vi "Byte Array to Supported Schemes.vi"(1 "Buffer":u8[](array[numeric])) -> (0 "Supported Schemes":T1[](array[typedef]))   [LabVIEW 2021, in "Field_RnD_Services_LIBSSH2_Toolkit.lvlib" / "Session.lvclass"]
doc: "Converts a byte array of comma-delimited string values into a list of supported authentication schemes by the remote SSH/SFTP server."
uses:
  Session.lvclass
  Session.lvclass/Session.ctl
  Type Definitions/User Authentication Schemes.ctl
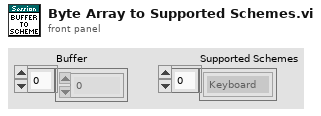
[diagram p1: front panel]
types:
  T1 = typedef "Field_RnD_Services_LIBSSH2_Toolkit.lvlib/Session.lvclass/User Authentication Schemes.ctl" = enum16{"Keyboard", "Password", "Public Key"}
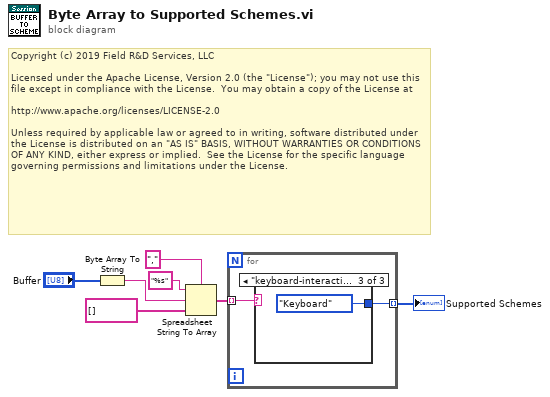
[diagram p0: block diagram]
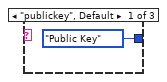
[diagram p2: hidden frame]
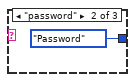
[diagram p3: hidden frame]
diagram:
  # "Copyright (c) 2019 Field R&D Services, LLC\n\nLicensed under the Apache License, Version 2.0 (the \"License\"); you may not use this file except in compliance with the License.  You may obtain a copy of the License at\n\nhttp://www.apache.org/licenses/LICENSE-2.0\n\nUnless required by applicable law or agreed to in writing, software distributed under the License is distributed on an \"AS IS\" BASIS, WITHOUT WARRANTIES OR CONDITIONS OF ANY KIND, either express or implied.  See the License for the specific language governing permissions and limitations under the License."
  n1 = Byte Array To String(unsigned byte array="Buffer") -> (string=w1:string)
  n2 = Spreadsheet String To Array(delimiter (Tab)=",", format string="%s", spreadsheet string=w1, array type (2D Dbl)=string[] []) -> (array=w5:string[])
  n3 = for {
    tunnel: w5 -> [w9] mode=indexing
    tunnel: [w8] -> w7 mode=indexing
    n4 = case shown="\"keyboard-interactive\"" w9 {
      tunnel: [User_Authentication_Schemes."Public Key" ("Scheme") User_Authentication_Schemes."Password" ("Scheme") User_Authentication_Schemes."Keyboard" ("Scheme")] -> w8
      frame "publickey", Default {
      }
      frame "password" {
      }
      frame "keyboard-interactive" {
      }
    }
  }
  "Supported Schemes" <- w7
